vi "ConvertTag__slk_tc.vi"(0 "tree control in":refnum<class "TreeControl.lvclass">, 5 "input tag (current tag)":string, 11 "error in (no error)":errorcluster, 12 "column # (0)":i32) -> (4 "tree control out":refnum<class "TreeControl.lvclass">, 6 "duplicated tag":string, 10 "text":string, 15 "error out":errorcluster)   [LabVIEW 2020, in "TreeControl.lvclass"]
doc: "Retrieves the text in column 0 assosciated with the Input Tag or if there is no input, the currently selected item. Ignores the call if no item is selected. Returns error code 1136 if an improper tag is input."
uses:
  Library/TreeControl.lvclass
  Library/TreeControl.lvclass/TreeControl.ctl
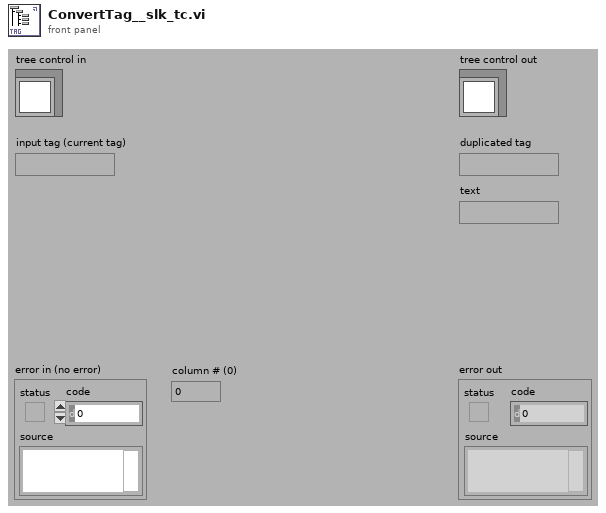
[diagram p1: front panel]
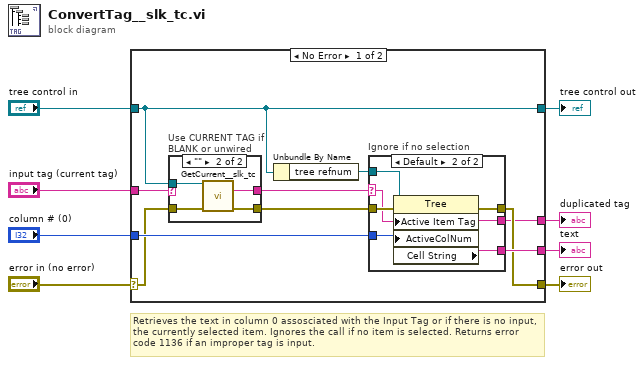
[diagram p0: block diagram]
diagram:
  # "Retrieves the text in column 0 assosciated with the Input Tag or if there is no input, the currently selected item. Ignores the call if no item is selected. Returns error code 1136 if an improper tag is input."
  n1 = case shown="No Error" "error in (no error)" {
    selector: "error in (no error)" -> [w13 w34]
    tunnel: [w12 w34] -> w7
    tunnel: [w11 w33] -> w5
    tunnel: "tree control in" -> [w11 w33]
    tunnel: "input tag (current tag)" -> [w18 _]
    tunnel: "column # (0)" -> [w15 _]
    tunnel: [w14 _] -> w2
    tunnel: [w9 _] -> w1
    frame No Error {
      n2 = case "Use CURRENT TAG if BLANK or unwired" shown="\"\"" w18 {
        selector: w18 -> [w28 _]
        tunnel: [w28 w32] -> w17
        tunnel: w11 -> [_ w31]
        tunnel: w13 -> [w27 w30]
        tunnel: [w27 w29] -> w16
        frame Default {
        }
        frame "" {
          n3 = call "GetCurrent__slk_tc.vi"("tree control in"=w31, "error in (no error)"=w30) -> ("current tag"=w32:string, "error out"=w29:errorcluster)  [unwired: 1 in, 11 out]
        }
      }
      n4 = Unbundle By Name(w11) -> ("tree refnum"=w10:refnum<vi>)
      n5 = case "Ignore if no selection" shown="Default" w17 {
        selector: w17 -> [w19 w21]
        tunnel: w16 -> [w20 w26]
        tunnel: w15 -> [_ w25]
        tunnel: [w20 w24] -> w12
        tunnel: [w19 w23] -> w14
        tunnel: w10 -> [_ w22]
        tunnel: [w19 w21] -> w9
        frame "" {
        }
        frame Default {
          n6 = property class="Tree"(reference=w22, error in=w26, "Active Item Tag"=w21, "ActiveColNum"=w25) -> (error out=w24:errorcluster, "Cell String"=w23:string)  [unwired: 1 out]
        }
      }
    }
    frame Error {
    }
  }
  "error out" <- w7
  "tree control out" <- w5
  "text" <- w2
  "duplicated tag" <- w1
